vi "WeldVsRad.vi"(8 "Outside":bool, 9 "BinSize (mm)":dbl, 10 "NumBins":dbl, 11 "Dists":cluster{dbl[]}[](array[cluster])) -> (3 "WeldVsRadius":dbl[](graph))   [LabVIEW 2014]
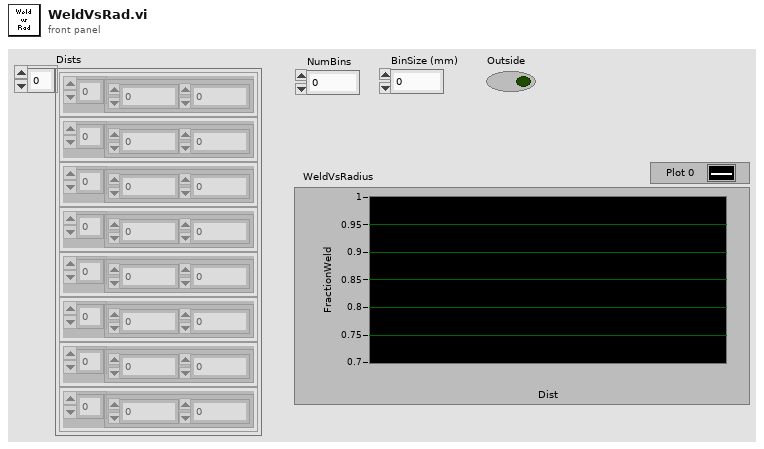
[diagram p1: front panel]
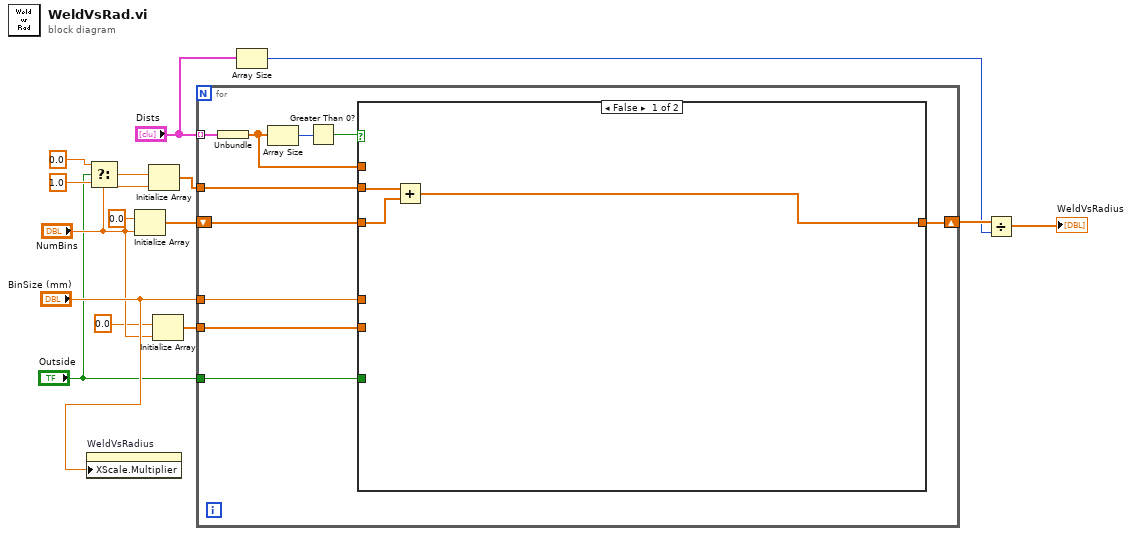
[diagram p0: block diagram]
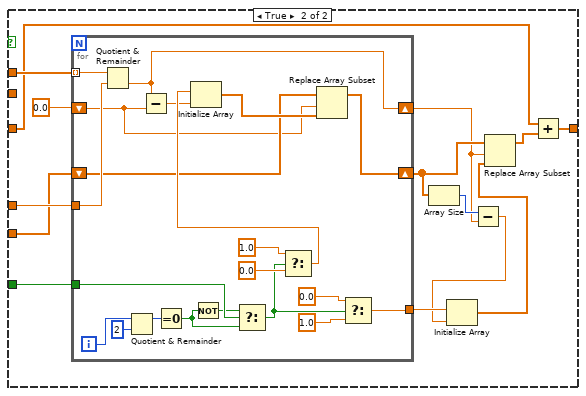
[diagram p2: hidden frame]
diagram:
  n1 = property on="WeldVsRadius" class="WFGraph (strict)"("XScale.Multiplier"="BinSize (mm)") -> ()  [unwired: 2 in, 2 out]
  n2 = Select(t=0.0 ("element"), s="Outside", f=1.0 ("element")) -> (s? t:f=w7:dbl)
  n3 = Initialize Array(0.0 ("element"), "NumBins") -> (w14:dbl[])
  n4 = Initialize Array(w7, "NumBins") -> (w3:dbl[])
  n5 = Initialize Array(0.0 ("element"), "NumBins") -> (w9:dbl[])
  n6 = for {
    tunnel: "Dists" -> [w25] mode=indexing
    shift-right: [w21] -> w13
    shift-left: w14 -> [w22]
    tunnel: "BinSize (mm)" -> [w19]
    tunnel: "Outside" -> [w18]
    tunnel: w9 -> [w17]
    tunnel: w3 -> [w16]
    n7 = Unbundle(w25) -> (w20:dbl[])
    n8 = Array Size(array=w20) -> (size(s)=w24:i32)
    n9 = Greater Than 0?(x=w24) -> (x > 0?=w23:bool)
    n10 = case shown="False" w23 {
      tunnel: w16 -> [w28 _]
      tunnel: w22 -> [w27 w37]
      tunnel: [w26 w38] -> w21
      tunnel: w20 -> [_ w42]
      tunnel: w19 -> [_ w41]
      tunnel: w18 -> [_ w40]
      tunnel: w17 -> [_ w36]
      frame False {
        n11 = Add(x=w28, y=w27) -> (x+y=w26:dbl[])
      }
      frame True {
        n12 = for {
          tunnel: w42 -> [w63] mode=indexing
          tunnel: w41 -> [w62]
          tunnel: w40 -> [w58]
          shift-right: [w54] -> w30
          shift-left: 0.0 -> [w49]
          shift-right: [w50] -> w31
          shift-left: w36 -> [w51]
          tunnel: [w43] -> w35
          i -> [w61]
          n13 = Quotient & Remainder(x=w63, y=w62) -> (floor(x/y)=w54:dbl)  [unwired: 1 out]
          n14 = Quotient & Remainder(x=w61, y=2) -> (x-y*floor(x/y)=w59:i32)  [unwired: 1 out]
          n15 = Subtract(x=w54, y=w49) -> (x-y=w53:dbl)
          n16 = Equal To 0?(x=w59) -> (x = 0?=w47:bool)
          n17 = Not(x=w47) -> (.not. x?=w48:bool)
          n18 = Select(t=w48, s=w58, f=w47) -> (s? t:f=w44:bool)
          n19 = Select(t=1.0, s=w44, f=0.0) -> (s? t:f=w55:dbl)
          n20 = Initialize Array(w55, w53) -> (w52:dbl[])
          n21 = Replace Array Subset(array=w51, new element=w52, index=w49) -> (w50:dbl[])
          n22 = Select(t=0.0, s=w44, f=1.0) -> (s? t:f=w43:dbl)
        }
        n23 = Array Size(array=w31) -> (size(s)=w34:i32)
        n24 = Subtract(x=w34, y=w30) -> (x-y=w33:dbl)
        n25 = Initialize Array(w35, w33) -> (w29:dbl[])
        n26 = Replace Array Subset(array=w31, new element=w29, index=w30) -> (w32:dbl[])
        n27 = Add(x=w37, y=w32) -> (x+y=w38:dbl[])
      }
    }
  }
  n28 = Array Size(array="Dists") -> (size(s)=w11:i32)
  n29 = Divide(x=w13, y=w11) -> (x/y=→"WeldVsRadius":dbl[])
